vi "NodeToGalvo.vi"(9 "nodeitem":i32, 10 "Index":dbl, 11 "Array":dbl[][](array[numeric])) -> (0 "AI out":refnum<k21>, 1 "AO out":refnum<k21>, 2 "element":dbl, 3 "Node":dbl[](array[numeric]))   [LabVIEW 2020]
uses:
  <resource>/objmgr/daqmx.rc
  <vilib>/DAQmx/create/channels.llb/DAQmx Create Channel (AO-Voltage-Basic).vi
  <vilib>/DAQmx/configure/timing.llb/DAQmx Timing (Sample Clock).vi
  <vilib>/DAQmx/write.llb/DAQmx Write (Analog 2D DBL NChan NSamp).vi
  <vilib>/DAQmx/create/channels.llb/DAQmx Create Channel (AI-Voltage-Basic).vi
panel:
  out "x/y":dbl[][](array[numeric])
  out "Y Offset":i32
  out "X Offset":i32
  out "Size":i32
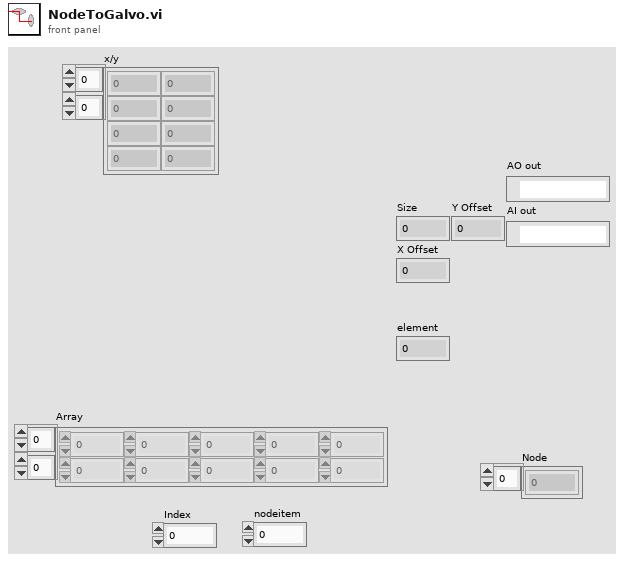
[diagram p1: front panel]
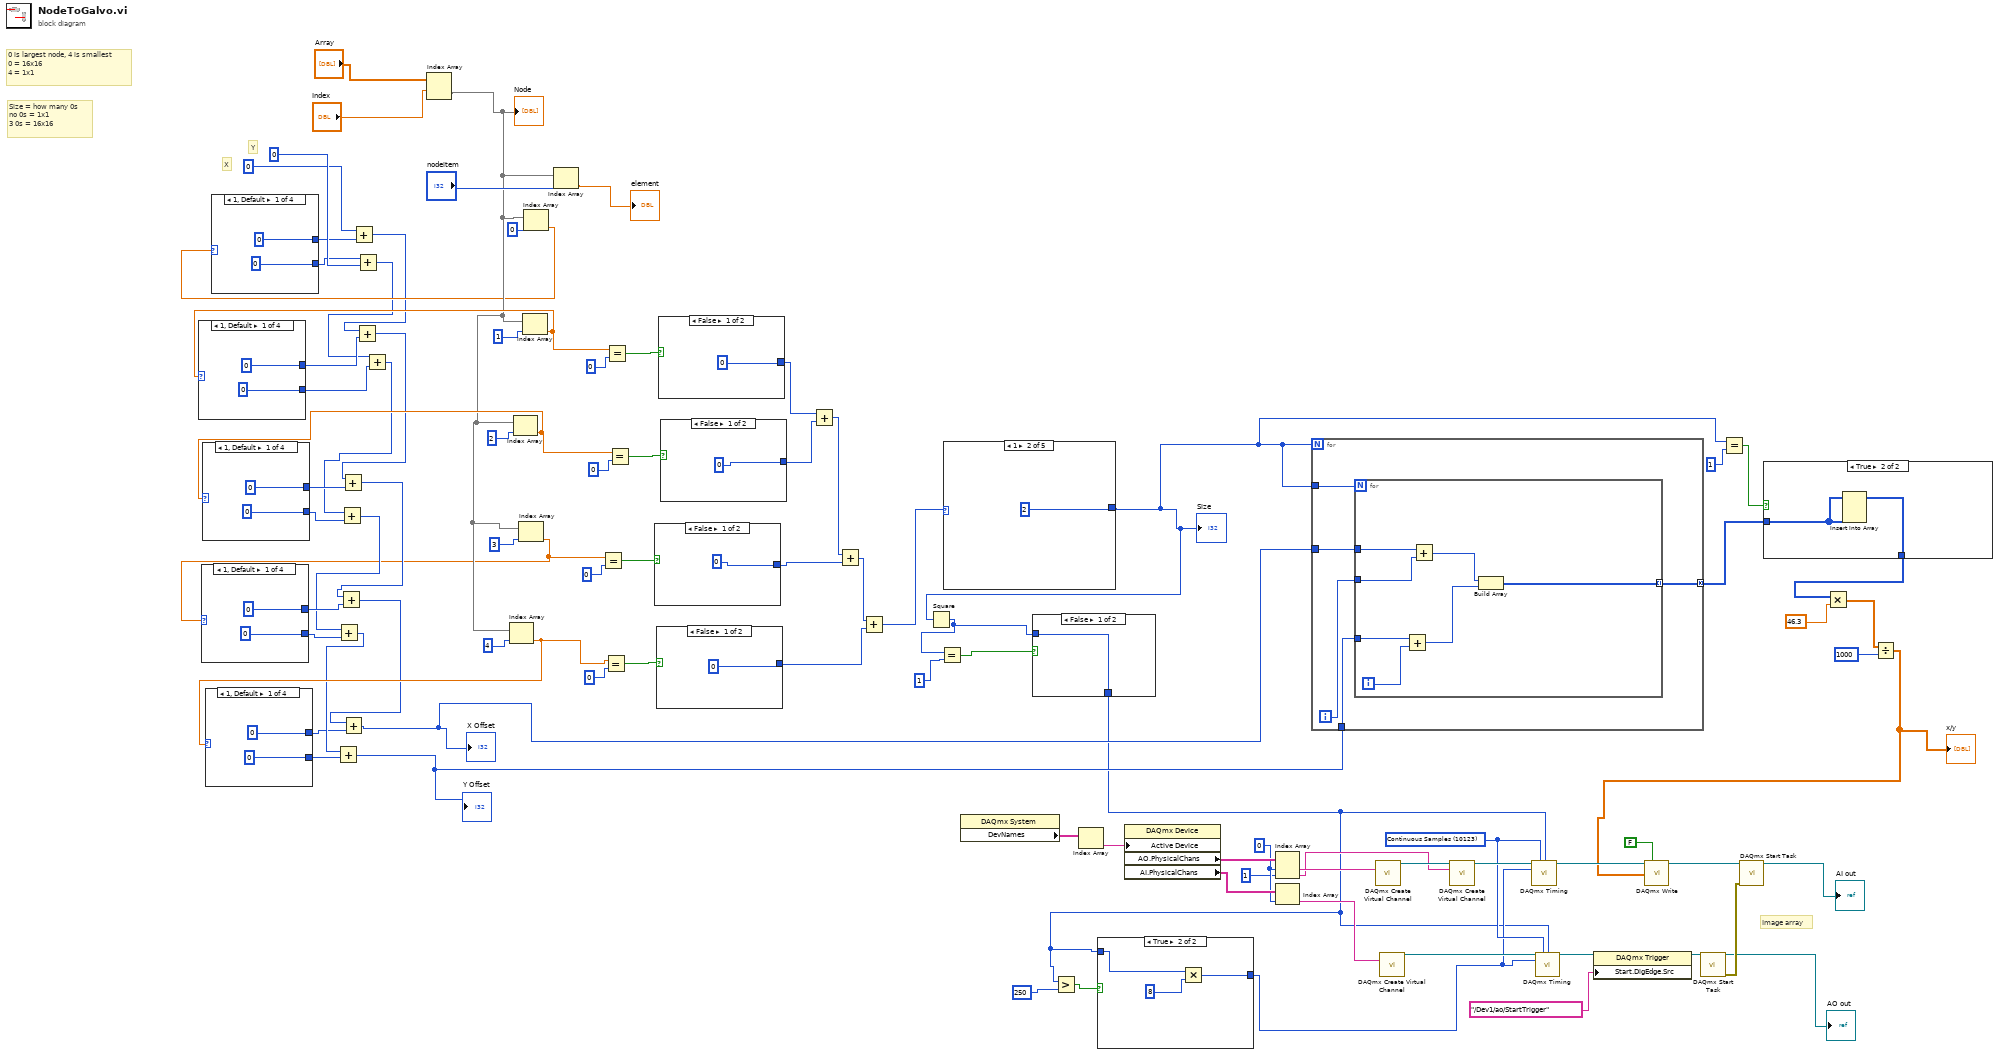
[diagram p0: block diagram]
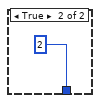
[diagram p2: hidden frame]
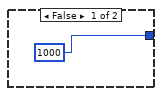
[diagram p4: hidden frame]
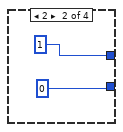
[diagram p5: hidden frame]
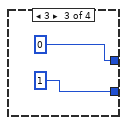
[diagram p6: hidden frame]
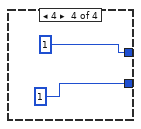
[diagram p7: hidden frame]
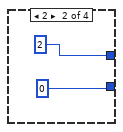
[diagram p8: hidden frame]
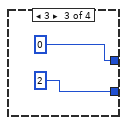
[diagram p9: hidden frame]
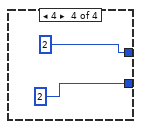
[diagram p10: hidden frame]
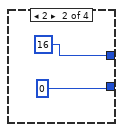
[diagram p11: hidden frame]
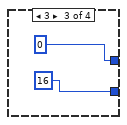
[diagram p12: hidden frame]
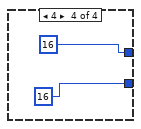
[diagram p13: hidden frame]
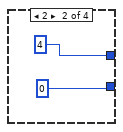
[diagram p14: hidden frame]
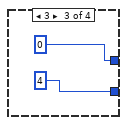
[diagram p15: hidden frame]
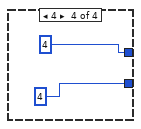
[diagram p16: hidden frame]
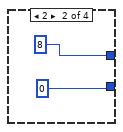
[diagram p17: hidden frame]
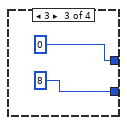
[diagram p18: hidden frame]
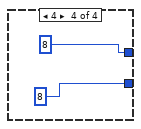
[diagram p19: hidden frame]
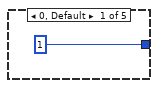
[diagram p20: hidden frame]
diagram:
  w23 = 10123 items=["Finite Samples"=10178, "Continuous Samples"=10123, "Hardware Timed Single Point"=12522] ("sample mode")
  w38 = 0 ("index")
  # "Image array"
  # "Y"
  # "X"
  # "Size = how many 0s\nno 0s = 1x1\n3 0s = 16x16"
  # "0 is largest node, 4 is smallest\n0 = 16x16\n4 = 1x1"
  n1 = Index Array(array="Array", index (row)="Index") -> (element=w64:dbl[])  [unwired: 1 in]
  "Node" <- w64
  n2 = Index Array(array=w64, index=4) -> (element=w61:dbl)
  n3 = case shown="1, Default" w61 {
    tunnel: [0 1 0 1] -> w44
    tunnel: [0 0 1 1] -> w43
    frame 1, Default {
    }
    frame 2 {
    }
    frame 3 {
    }
    frame 4 {
    }
  }
  n4 = Index Array(array=w64, index=2) -> (element=w65:dbl)
  n5 = case shown="1, Default" w65 {
    tunnel: [0 4 0 4] -> w53
    tunnel: [0 0 4 4] -> w51
    frame 1, Default {
    }
    frame 2 {
    }
    frame 3 {
    }
    frame 4 {
    }
  }
  n6 = Index Array(array=w64, index=3) -> (element=w14:dbl)
  n7 = case shown="1, Default" w14 {
    tunnel: [0 2 0 2] -> w49
    tunnel: [0 0 2 2] -> w48
    frame 1, Default {
    }
    frame 2 {
    }
    frame 3 {
    }
    frame 4 {
    }
  }
  n8 = Index Array(array=w64, index=1) -> (element=w68:dbl)
  n9 = case shown="1, Default" w68 {
    tunnel: [0 8 0 8] -> w66
    tunnel: [0 0 8 8] -> w67
    frame 1, Default {
    }
    frame 2 {
    }
    frame 3 {
    }
    frame 4 {
    }
  }
  n10 = Index Array(array=w64, index=0) -> (element=w62:dbl)
  n11 = case shown="1, Default" w62 {
    tunnel: [0 16 0 16] -> w58
    tunnel: [0 0 16 16] -> w57
    frame 1, Default {
    }
    frame 2 {
    }
    frame 3 {
    }
    frame 4 {
    }
  }
  n12 = Add(x=0, y=w58) -> (x+y=w56:i32)
  n13 = Add(x=w56, y=w66) -> (x+y=w54:i32)
  n14 = Add(x=w54, y=w53) -> (x+y=w50:i32)
  n15 = Add(x=w50, y=w49) -> (x+y=w46:i32)
  n16 = Add(x=w46, y=w44) -> (x+y=w19:i32)
  "X Offset" <- w19
  n17 = Add(x=w57, y=0) -> (x+y=w55:i32)
  n18 = Add(x=w55, y=w67) -> (x+y=w52:i32)
  n19 = Add(x=w52, y=w51) -> (x+y=w47:i32)
  n20 = Add(x=w47, y=w48) -> (x+y=w45:i32)
  n21 = Add(x=w45, y=w43) -> (x+y=w20:i32)
  "Y Offset" <- w20
  n22 = Index Array(array=w64, index="nodeitem") -> (element=→"element":dbl)
  n23 = Equal?(x=w14, y=0) -> (x = y?=w79:bool)
  n24 = Equal?(x=w61, y=0) -> (x = y?=w76:bool)
  n25 = Equal?(x=w68, y=0) -> (x = y?=w85:bool)
  n26 = Equal?(x=w65, y=0) -> (x = y?=w82:bool)
  n27 = case shown="False" w79 {
    tunnel: [0 1] -> w71
    frame False {
    }
    frame True {
    }
  }
  n28 = case shown="False" w76 {
    tunnel: [0 1] -> w70
    frame False {
    }
    frame True {
    }
  }
  n29 = case shown="False" w85 {
    tunnel: [0 1] -> w74
    frame False {
    }
    frame True {
    }
  }
  n30 = case shown="False" w82 {
    tunnel: [0 1] -> w73
    frame False {
    }
    frame True {
    }
  }
  n31 = Add(x=w74, y=w73) -> (x+y=w72:i32)
  n32 = Add(x=w72, y=w71) -> (x+y=w69:i32)
  n33 = Add(x=w69, y=w70) -> (x+y=w10:i32)
  n34 = case shown="1" w10 {
    tunnel: [1 2 4 8 16] -> w4
    frame 0, Default {
    }
    frame 1 {
    }
    frame 2 {
    }
    frame 3 {
    }
    frame 4 {
    }
  }
  "Size" <- w4
  n35 = Square(x=w4) -> (x^2=w2:i32)
  n36 = Equal?(x=w2, y=1) -> (x = y?=w3:bool)
  n37 = property class="DAQmx System"() -> ("DevNames"=w42:tag[])  [unwired: 2 in, 2 out]
  n38 = case shown="False" w3 {
    tunnel: w2 -> [w144 _]
    tunnel: [w144 2] -> w1
    frame False {
    }
    frame True {
    }
  }
  n39 = Greater?(x=w1, y=250) -> (0:w13:bool)
  n40 = Index Array(array=w42) -> (element=w41:tag)  [unwired: 1 in]
  n41 = case shown="True" w13 {
    tunnel: w1 -> [_ w148]
    tunnel: [1000 w147] -> w11
    frame False {
    }
    frame True {
      n42 = Multiply(x=w148, y=8) -> (x*y=w147:i32)
    }
  }
  n43 = property class="DAQmx Device"("Active Device"=w41) -> ("AO.PhysicalChans"=w40:tag[], "AI.PhysicalChans"=w39:tag[])  [unwired: 2 in, 2 out]
  n44 = Index Array(array=w40, index #1=w38, index #2=1 ("index")) -> (element #1=w36:tag, element #2=w34:tag)
  n45 = Index Array(array=w39, index=w38) -> (element=w33:tag)
  n46 = for {
    N: w4 -> [_]
    tunnel: w4 -> [w154]
    tunnel: [w152] -> w7 mode=concatenating
    tunnel: w20 -> [w151]
    tunnel: w19 -> [w150]
    i -> [w153]
    n47 = for {
      N: w154 -> [_]
      tunnel: w153 -> [w156]
      tunnel: [w161] -> w152 mode=indexing
      tunnel: w151 -> [w160]
      tunnel: w150 -> [w157]
      i -> [w159]
      n48 = Add(x=w160, y=w159) -> (x+y=w158:i32)
      n49 = Add(x=w157, y=w156) -> (x+y=w155:i32)
      n50 = Build Array(w155, w158) -> (w161:i32[])
    }
  }
  n51 = call-poly <vilib>:"DAQmx Create Virtual Channel.vi"("physical channels"=w36) -> ("task out"=w35:refnum<k21>)  [unwired: 13 in, 1 out]
  n52 = call-poly <vilib>:"DAQmx Create Virtual Channel.vi"("physical channels"=w33) -> ("task out"=w32:refnum<k21>)  [unwired: 13 in, 1 out]
  n53 = call-poly <vilib>:"DAQmx Create Virtual Channel.vi"("task in"=w35, "physical channels"=w34) -> ("task out"=w31:refnum<k21>)  [unwired: 12 in, 1 out]
  n54 = call-poly <vilib>:"DAQmx Timing.vi"("task/channels in"=w31, "sample mode"=w23, "samples per channel"=w1, "rate"=w11) -> ("task out"=w26:refnum<k21>)  [unwired: 10 in, 1 out]
  n55 = call-poly <vilib>:"DAQmx Timing.vi"("task/channels in"=w32, "sample mode"=w23, "samples per channel"=w1, "rate"=w11) -> ("task out"=w30:refnum<k21>)  [unwired: 10 in, 1 out]
  n56 = property class="DAQmx Trigger"(reference=w30, "Start.DigEdge.Src"=tag "/Dev1/ao/StartTrigger") -> (reference out=w28:refnum<k21>)  [unwired: 1 in, 1 out]
  n57 = call <vilib>:"DAQmx Start Task.vi"("task/channels in"=w28) -> ("task out"=→"AO out":refnum<k21>, "error out"=w27:errorcluster)  [unwired: 13 in]
  n58 = Equal?(x=w4, y=1) -> (x = y?=w8:bool)
  n59 = case shown="True" w8 {
    tunnel: w7 -> [w162 w164]
    tunnel: [w162 w163] -> w6
    frame False {
    }
    frame True {
      n60 = Insert Into Array(array=w164, new element=w164) -> (w163:i32[][])  [unwired: 2 in]
    }
  }
  n61 = Multiply(x=w6, y=46.3) -> (x*y=w17:dbl[][])
  n62 = Divide(x=w17, y=1000) -> (x/y=w15:dbl[][])
  "x/y" <- w15
  n63 = call-poly <vilib>:"DAQmx Write.vi"("task/channels in"=w26, "auto start"=FALSE, "data"=w15) -> ("task out"=w25:refnum<k21>)  [unwired: 10 in, 2 out]
  n64 = call <vilib>:"DAQmx Start Task.vi"("task/channels in"=w25, "error in"=w27) -> ("task out"=→"AI out":refnum<k21>)  [unwired: 12 in, 1 out]
